vi "Param Test.vi"() -> ()   [LabVIEW 2020]
uses:
  g_ar_toolkit.capture/CameraStream/Camera Automatic Parameter Mode.ctl
  g_ar_toolkit.capture/CameraStream/Camera Parameter Information.ctl
  g_ar_toolkit.capture/CameraStream/CameraStream.lvclass/CameraStream.ctl
  g_ar_toolkit.image/CreateEmptyImageARGB.vi
  g_ar_toolkit.image/DrawImageToPictureARGB.vi
  7a086690-3a27-4eb0-92c0-07a8b9dc1a9d.vi
  bd8472f0-af5e-3fd8-803b-1528c88fa43f.vi
  g_ar_toolkit.capture/CameraStream/Get Focus Parameter Info.vi
  g_ar_toolkit.capture/CameraStream/Get Focus Parameter.vi
  g_ar_toolkit.capture/CameraStream/Get Zoom Parameter Info.vi
  g_ar_toolkit.capture/CameraStream/Get Zoom Parameter.vi
  g_ar_toolkit.capture/CameraStream/Get White Balance Parameter Info.vi
  g_ar_toolkit.capture/CameraStream/Get White Balance Parameter.vi
  g_ar_toolkit.capture/CameraStream/Get Brightenss Parameter Info.vi
  g_ar_toolkit.capture/CameraStream/Get Brightenss Parameter.vi
  g_ar_toolkit.capture/CameraStream/Get Contrast Parameter Info.vi
  g_ar_toolkit.capture/CameraStream/Get Contrast Parameter.vi
  g_ar_toolkit.capture/CameraStream/Get Saturation Parameter Info.vi
  g_ar_toolkit.capture/CameraStream/Get Saturation Parameter.vi
  g_ar_toolkit.capture/CameraStream/Get Gamma Parameter Info.vi
  g_ar_toolkit.capture/CameraStream/Get Gamma Parameter.vi
  g_ar_toolkit.capture/CameraStream/Get Hue Parameter Info.vi
  g_ar_toolkit.capture/CameraStream/Get Hue Parameter.vi
  g_ar_toolkit.capture/CameraStream/Get Sharpness Parameter Info.vi
  g_ar_toolkit.capture/CameraStream/Get Sharpness Parameter.vi
  g_ar_toolkit.capture/CameraStream/Get Backlight Compensation Parameter Info.vi
  g_ar_toolkit.capture/CameraStream/Get Backlight Compensation Parameter.vi
  g_ar_toolkit.capture/CameraStream/Get Powerline Frequency Parameter Info.vi
  g_ar_toolkit.capture/CameraStream/Get Powerline Frequency Parameter.vi
  g_ar_toolkit.capture/CameraStream/Get Exposure Parameter Info.vi
  g_ar_toolkit.capture/CameraStream/Get Exposure Parameter.vi
  g_ar_toolkit.capture/CameraStream/Get Automatic Focus Mode.vi
  g_ar_toolkit.capture/CameraStream/Get Automatic White Balance Mode.vi
  g_ar_toolkit.capture/CameraStream/Get Automatic Gain Mode.vi
  g_ar_toolkit.capture/CameraStream/Get Automatic Exposure Mode.vi
  g_ar_toolkit.capture/CameraStream/Get Gain Parameter Info.vi
  g_ar_toolkit.capture/CameraStream/Get Gain Parameter.vi
  g_ar_toolkit.capture/CameraStream/Set Focus Parameter.vi
  g_ar_toolkit.capture/CameraStream/Set Zoom Parameter.vi
  g_ar_toolkit.capture/CameraStream/Set White Balance Parameter.vi
  g_ar_toolkit.capture/CameraStream/Set Gain Parameter.vi
  g_ar_toolkit.capture/CameraStream/Set Brightenss Parameter.vi
  g_ar_toolkit.capture/CameraStream/Set Contrast Parameter.vi
  g_ar_toolkit.capture/CameraStream/Set Saturation Parameter.vi
  g_ar_toolkit.capture/CameraStream/Set Gamma Parameter.vi
  g_ar_toolkit.capture/CameraStream/Set Hue Parameter.vi
  g_ar_toolkit.capture/CameraStream/Set Sharpness Parameter.vi
  g_ar_toolkit.capture/CameraStream/Set Backlight Compensation Parameter.vi
  g_ar_toolkit.capture/CameraStream/Set Powerline Frequency Parameter.vi
  g_ar_toolkit.capture/CameraStream/Set Exposure Parameter.vi
  g_ar_toolkit.capture/CameraStream/Set Automatic Focus Mode.vi.vi
  g_ar_toolkit.capture/CameraStream/Set Automatic White Balance Mode.vi
  g_ar_toolkit.capture/CameraStream/Set Automatic Gain Mode.vi.vi
  g_ar_toolkit.capture/CameraStream/Set Automatic Exposure Mode.vi.vi
  g_ar_toolkit.image/CreateEmptyImageARGB.vi/3321fa97-f432-4e1e-8db9-a0df79aed21b.vi
  g_ar_toolkit.image/DrawImageToPictureARGB.vi/8cd07b1b-062e-4fe4-9e87-2eb3dc89fe0e.vi
  g_ar_toolkit.capture/CameraStream/GetParameterInfo.vi
  g_ar_toolkit.capture/CameraStream/GetParameter.vi
  g_ar_toolkit.capture/CameraStream/GetAutomaticParameterMode.vi
  g_ar_toolkit.capture/CameraStream/SetParameter.vi
  g_ar_toolkit.capture/CameraStream/SetAutomaticParameterMode.vi
  g_ar_toolkit.image/ARGBColourToU32.vi
  <vilib>/Utility/error.llb/Error Cluster From Error Code.vi
  g_ar_toolkit.capture/CameraStream/CameraStream.lvclass
  g_ar_toolkit.capture/CameraManager/CameraManager.lvclass
  g_ar_toolkit.image/g_ar_toolkit.image.lvlib
panel:
  in  "Start/Stop":bool
  in  "Format":string(combo)
  in  "Source":string(combo)
  in  "Enumerate":bool
  in  "Erase":bool
  in  "Picture Zoom":dbl=1.0 min=0.0001 max=10.0 step=0.1
  out "Array":T2(array[cluster])
  in  "Automatic Parameter Mode":T3
  out "Array 2":T4(array[cluster])
  in  "Auto Parameter":T5(ring)
  out "Set Value":i32
  in  "enum":T6(ring)
  in  "Dial":i32(knob) step=1 scale=2800.0..6500.0
  out "2D Picture":picture
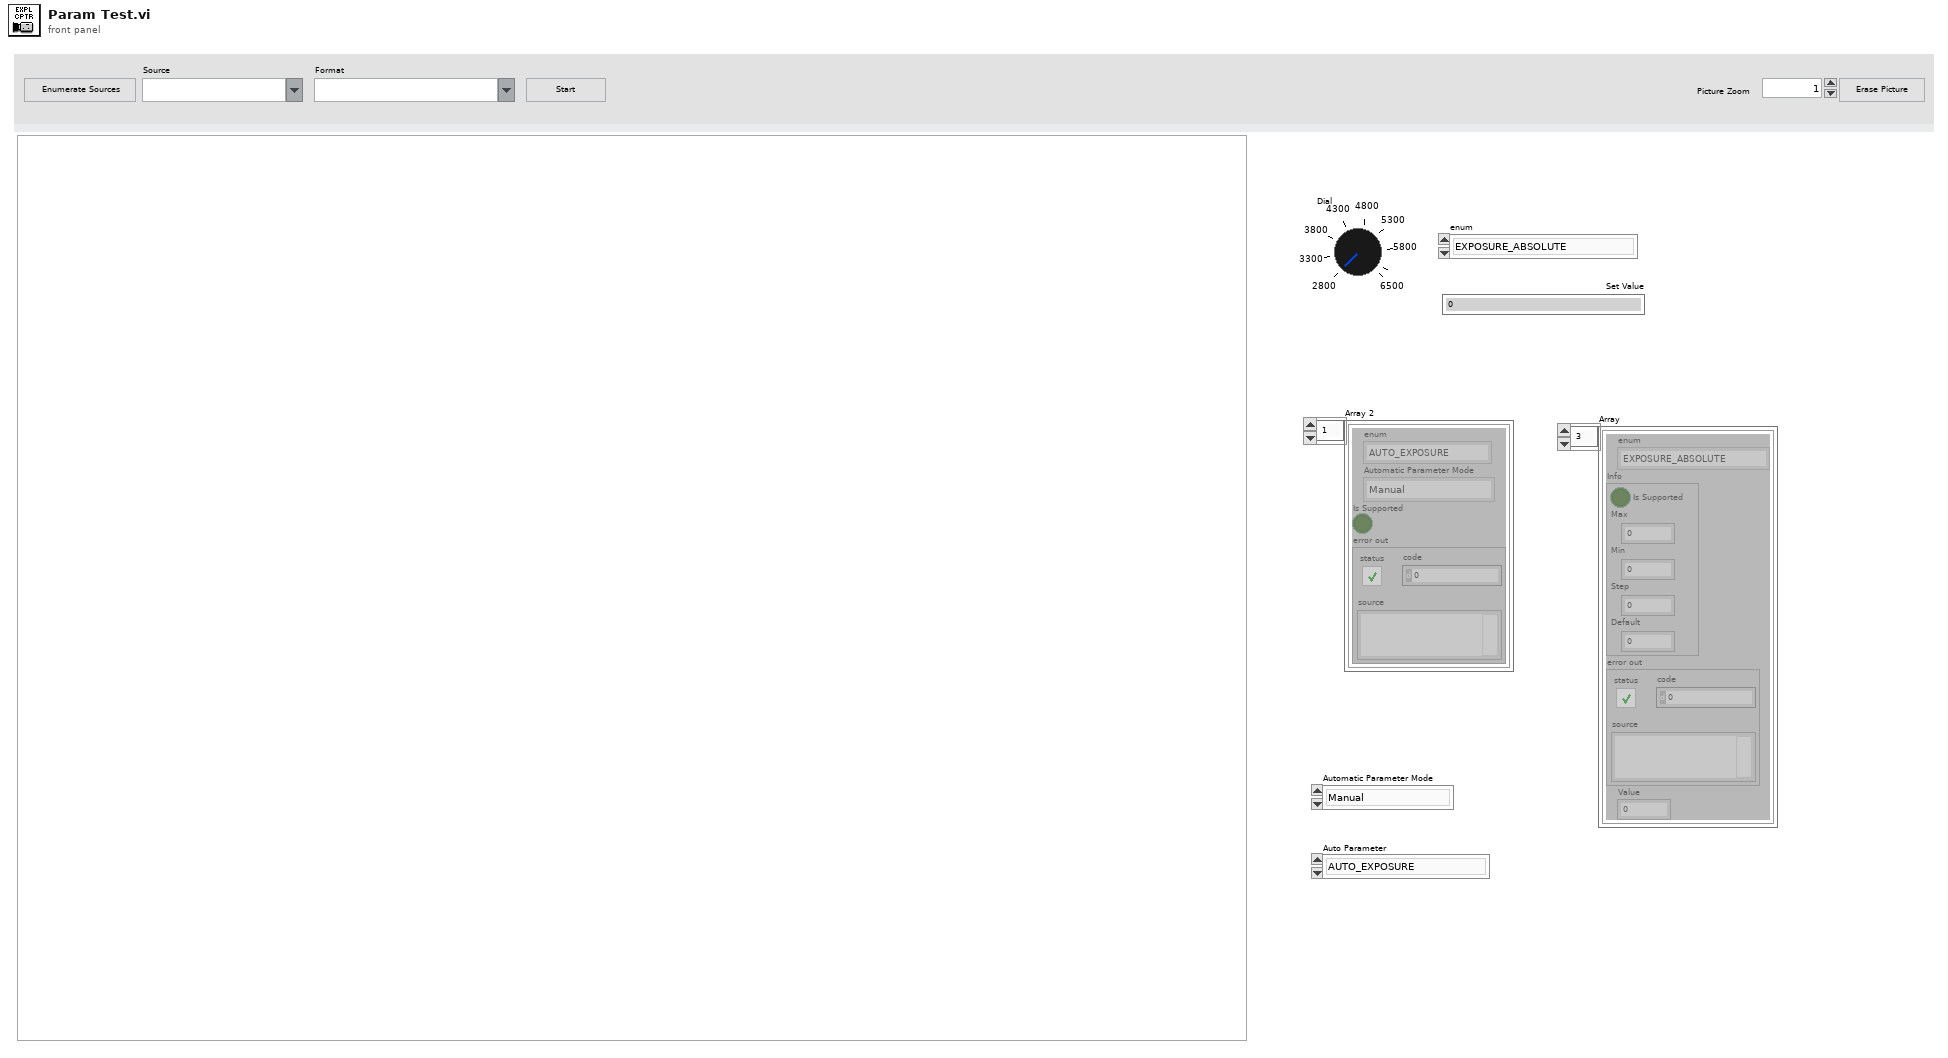
[diagram p1: front panel]
types:
  T1 = typedef "g_ar_toolkit.capture.lvlib/CameraStream.lvclass/Camera Parameter Information.ctl" = cluster{"Is Supported":bool, "Max":i32, "Min":i32, "Step":i32, "Default":i32}
  T2 = cluster{"enum":enum8{"EXPOSURE_ABSOLUTE", "FOCUS_ABSOLUTE", "ZOOM_ABSOLUTE", "WHITE_BALANCE_TEMPERATURE", "BRIGHTNESS", "CONTRAST", "SATURATION", "GAMMA", "HUE", "SHARPNESS", "BACKLIGHT_COMPENSATION", "POWER_LINE_FREQUENCY"}, "Info":T1, "error out":errorcluster, "Value":i32}[]
  T3 = typedef "g_ar_toolkit.capture.lvlib/CameraStream.lvclass/Camera Automatic Parameter Mode.ctl" = enum16{"Manual", "Automatic"}
  T4 = cluster{"enum":enum16{"AUTO_EXPOSURE", "AUTO_FOCUS", "AUTO_WHITEBALANCE", "AUTO_GAIN"}, "Automatic Parameter Mode":T3, "Is Supported":bool, "error out":errorcluster}[]
  T5 = enum16{"AUTO_EXPOSURE", "AUTO_FOCUS", "AUTO_WHITEBALANCE", "AUTO_GAIN"}
  T6 = enum8{"EXPOSURE_ABSOLUTE", "FOCUS_ABSOLUTE", "ZOOM_ABSOLUTE", "GAIN", "WHITE_BALANCE_TEMPERATURE", "BRIGHTNESS", "CONTRAST", "SATURATION", "GAMMA", "HUE", "SHARPNESS", "BACKLIGHT_COMPENSATION", "POWER_LINE_FREQUENCY"}
  T7 = enum8{"Enabled", "Disabled", "Disabled and Grayed Out"}
  T8 = enum8{"EXPOSURE_ABSOLUTE", "FOCUS_ABSOLUTE", "ZOOM_ABSOLUTE", "WHITE_BALANCE_TEMPERATURE", "BRIGHTNESS", "CONTRAST", "SATURATION", "GAMMA", "HUE", "SHARPNESS", "BACKLIGHT_COMPENSATION", "POWER_LINE_FREQUENCY"}
  T9 = typedef "g_ar_toolkit.capture.lvlib/CameraManager.lvclass/Device Enumeration.ctl" = cluster{"Name":string, "Streams":set{T10}}
  T10 = typedef "g_ar_toolkit.capture.lvlib/CameraManager.lvclass/Stream Parameters.ctl" = cluster{"Width":u16, "Height":u16, "FPS":u8}
  T11 = enum8{"EXPOSURE_ABSOLUTE", "FOCUS_ABSOLUTE", "ZOOM_ABSOLUTE", "WHITE_BALANCE_TEMPERATURE", "BRIGHTNESS", "CONTRAST", "SATURATION", "GAMMA", "HUE", "SHARPNESS", "BACKLIGHT_COMPENSATION", "POWER_LINE_FREQUENCY"}[]
  T12 = cluster{"enum":enum8{"EXPOSURE_ABSOLUTE", "FOCUS_ABSOLUTE", "ZOOM_ABSOLUTE", "WHITE_BALANCE_TEMPERATURE", "BRIGHTNESS", "CONTRAST", "SATURATION", "GAMMA", "HUE", "SHARPNESS", "BACKLIGHT_COMPENSATION", "POWER_LINE_FREQUENCY"}, "Info":T1, "error out":errorcluster, "Value":i32}
  T13 = enum16{"AUTO_EXPOSURE", "AUTO_FOCUS", "AUTO_WHITEBALANCE", "AUTO_GAIN"}[]
  T14 = cluster{"enum":enum16{"AUTO_EXPOSURE", "AUTO_FOCUS", "AUTO_WHITEBALANCE", "AUTO_GAIN"}, "Automatic Parameter Mode":T3, "Is Supported":bool, "error out":errorcluster}
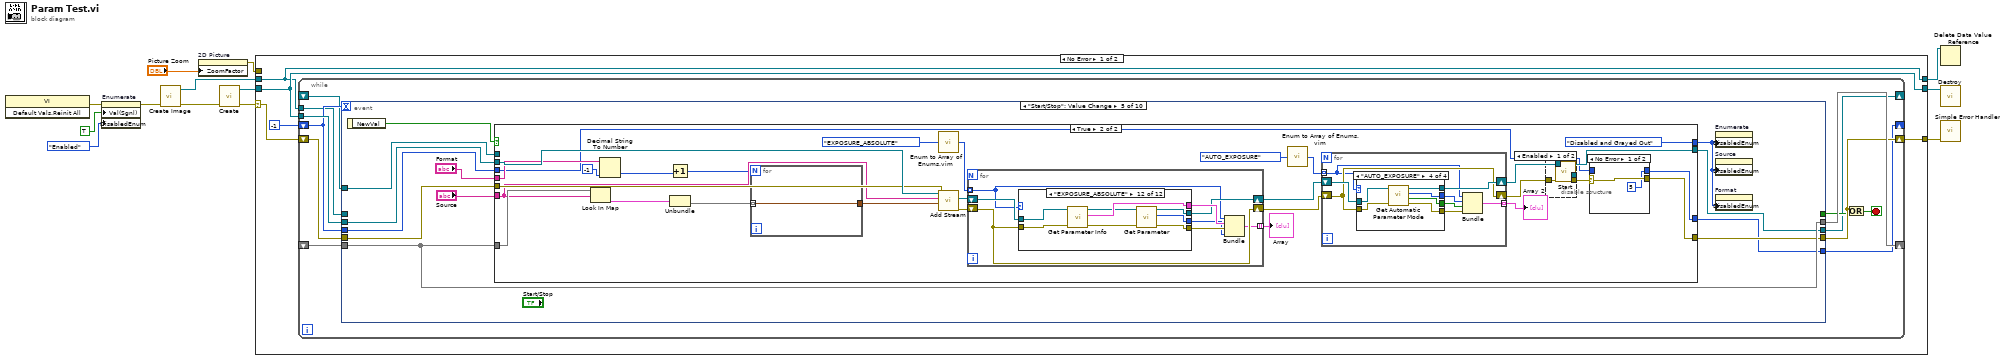
[diagram p0: block diagram]
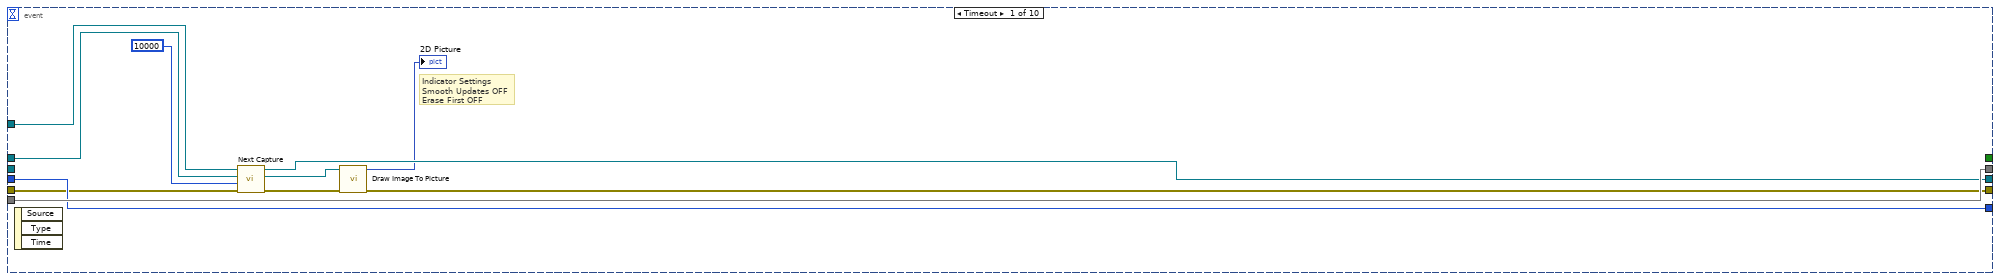
[diagram p2: hidden frame]
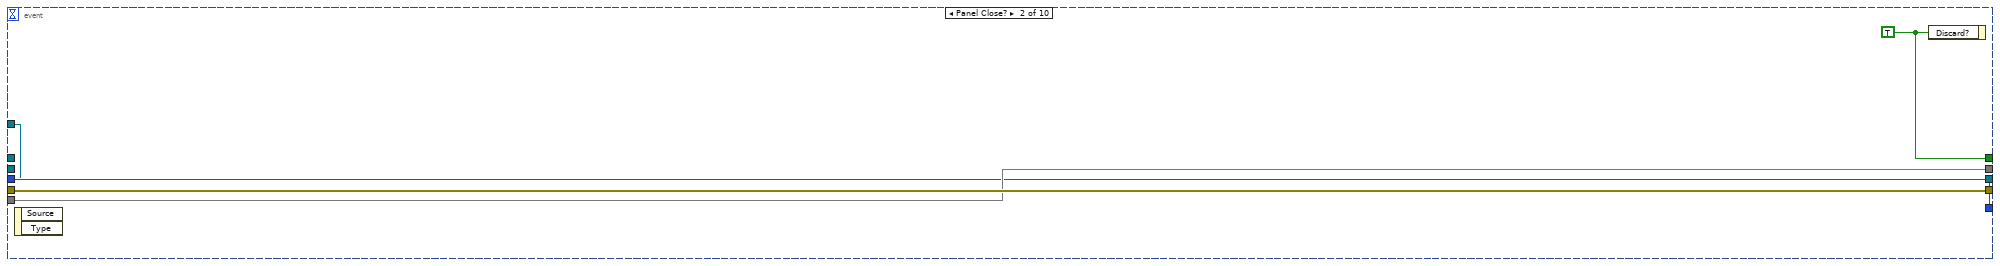
[diagram p3: hidden frame]
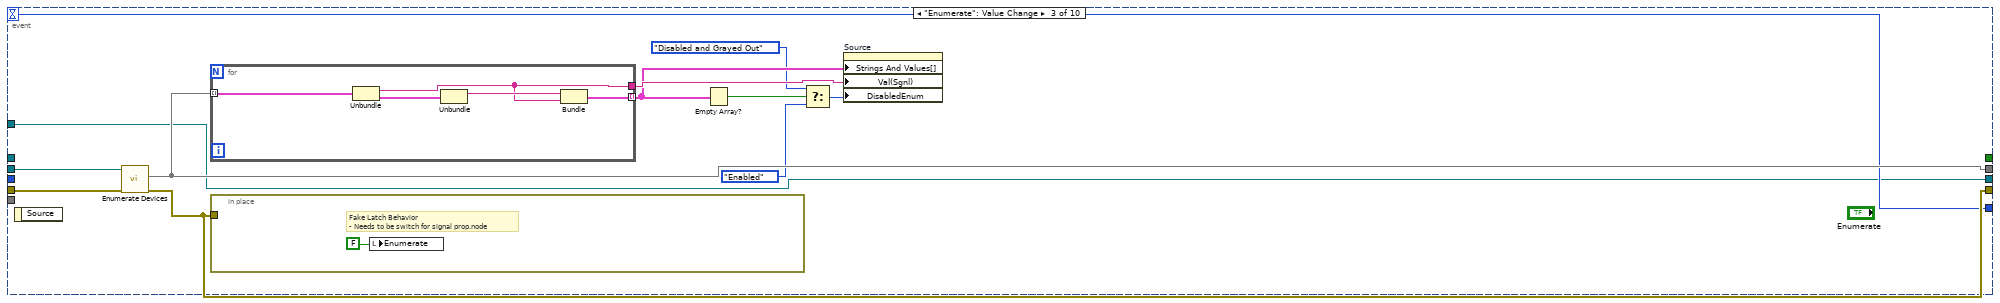
[diagram p4: hidden frame]
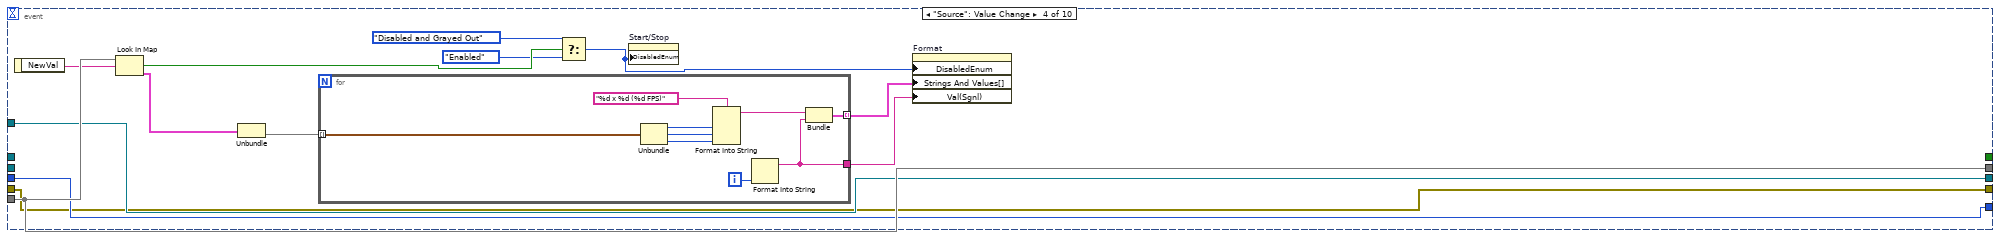
[diagram p5: hidden frame]
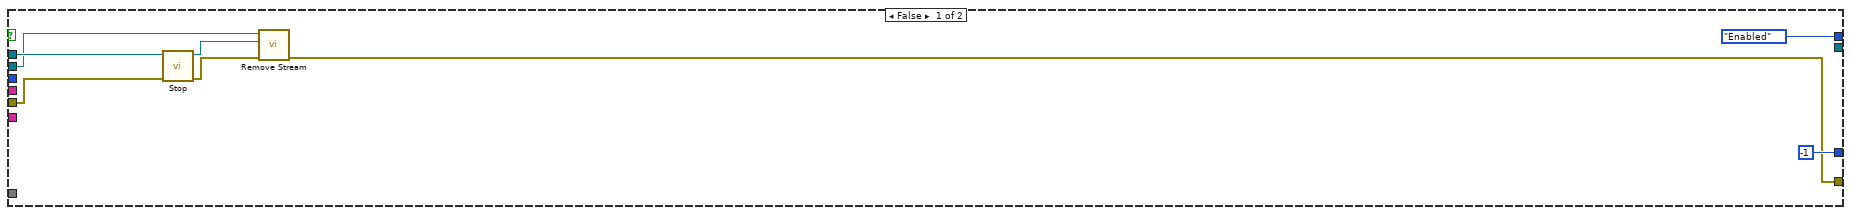
[diagram p6: hidden frame]
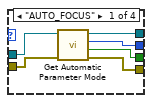
[diagram p8: hidden frame]
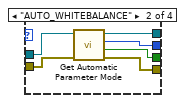
[diagram p9: hidden frame]
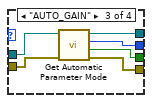
[diagram p10: hidden frame]
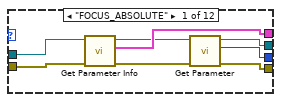
[diagram p11: hidden frame]
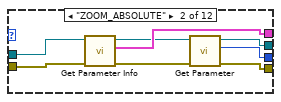
[diagram p12: hidden frame]
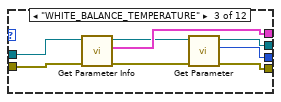
[diagram p13: hidden frame]
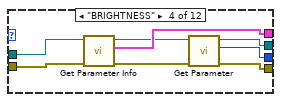
[diagram p14: hidden frame]
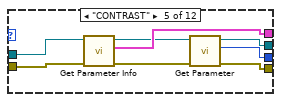
[diagram p15: hidden frame]
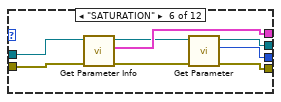
[diagram p16: hidden frame]
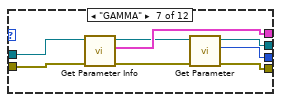
[diagram p17: hidden frame]
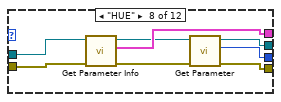
[diagram p18: hidden frame]
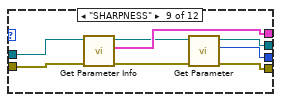
[diagram p19: hidden frame]
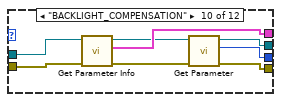
[diagram p20: hidden frame]
diagram:
  n1 = invoke class="VI" method="Default Vals.Reinit All"() -> (error out=w5:errorcluster)  [unwired: 3 in, 2 out]
  n2 = property on="Enumerate" class="Bool (strict)"(error in=w5, "Val(Sgnl)"=TRUE ("Value (Signaling)"), "DisabledEnum"=T7."Enabled" ("Disabled")) -> (error out=w1:errorcluster)  [unwired: 1 in, 1 out]
  n3 = call-poly "Create Image.vi"("error in (no error)"=w1) -> ("error out"=w4:errorcluster, "New ARGB Image"=w10:refnum<data-value>)  [unwired: 9 in]
  n4 = property on="2D Picture" class="Pict"("ZoomFactor"="Picture Zoom") -> (error out=w9:errorcluster)  [unwired: 2 in, 1 out]
  n5 = call "Create.vi"("error in (no error)"=w4) -> ("error out"=w13:errorcluster, "CameraManager"=w2:refnum<data-value>)  [unwired: 9 in]
  n6 = case shown="No Error" w13 {
    selector: w13 -> [w18 w564]
    tunnel: w2 -> [w17 w566]
    tunnel: [w17 w566] -> w12
    tunnel: w10 -> [w15 w565]
    tunnel: w9 -> [_ _]
    tunnel: [w15 w565] -> w7
    tunnel: [w14 w564] -> w6
    frame No Error {
      n7 = while {
        tunnel: w17 -> [w30]
        shift-right: [w28] -> _
        shift-left: _ -> [w27]
        shift-right: [w26] -> w14
        shift-left: w18 -> [w29]
        shift-right: [w23] -> _
        shift-left: -1 -> [w22]
        shift-right: [w21] -> _
        shift-left: _ -> [w20]
        tunnel: w15 -> [w19]
        stop <- w25 stop-if-true
        n8 = event shown="[4] \"Start/Stop\": Value Change" {
          selector: _ -> [_ _ _ _ _ _ _ _ _ _]
          dyn-events: _ -> [_ _ _ _ _ _ _ _ _ _]
          timeout: w22 -> [_ _ w53 _ _ _ _ _ _ _]
          tunnel: w30 -> [_ _ w58 _ w94 _ _ _ _ _]
          tunnel: w29 -> [w33 w45 w57 w65 w95 w287 w442 w527 w554 w560]
          tunnel: [w41 w44 w56 w77 w93 w299 w446 w532 w557 w558] -> w28
          tunnel: w27 -> [w41 w44 _ w77 w93 w299 w446 w532 w557 w558]
          tunnel: [w32 w45 w54 w65 w92 w289 w441 w528 w554 w559] -> w26
          tunnel: [_ w46 _ _ _ _ _ _ _ _] -> w24
          tunnel: [w40 w43 w53 w67 w89 w298 w445 w531 w556 w563] -> w23
          tunnel: w22 -> [w40 w43 _ w67 w90 w298 w445 w531 w556 w563]
          tunnel: [w38 w42 w52 w66 w91 w290 w443 w529 w555 w562] -> w21
          tunnel: w20 -> [w39 w42 w52 w66 w88 w288 w444 w530 w555 w562]
          tunnel: w19 -> [w37 _ _ _ _ _ _ _ _ _]
          event Timeout {
            # "Indicator Settings\nSmooth Updates OFF\nErase First OFF"
            n9 = event-data() -> ()  [unwired: 1 in, 3 out]
            n10 = call "Next Capture.vi"("error in (no error)"=w33, "timeout (ms)"=u16 10000, "ARGB Image Destination"=w37, "Stream"=w39) -> ("error out"=w34:errorcluster, "ARGB Image (duplicate)"=w35:refnum<data-value>, "Stream (duplicate)"=w38:refnum<data-value>)  [unwired: 5 in]
            n11 = call-poly "Draw Image To Picture.vi"("error in (no error)"=w34, "ARGB Image Source"=w35) -> ("error out"=w32:errorcluster, "Picture"=→"2D Picture":picture)  [unwired: 8 in]
          }
          event Panel Close? {
            w46 = TRUE ("Discard?")
            n12 = event-data() -> ()  [unwired: 1 in, 2 out]
            n13 = event-data("Discard?"=w46) -> ()  [unwired: 1 in, 1 out]
          }
          event "Enumerate": Value Change {
            n14 = event-data() -> ()  [unwired: 1 in, 1 out]
            n15 = call "Enumerate Devices.vi"("error in (no error)"=w57, "CameraManager"=w58) -> ("error out"=w54:errorcluster, "Devices"=w56:map{string, T9})  [unwired: 7 in, 1 out]
            n16 = for {
              tunnel: w56 -> [w64] mode=indexing
              tunnel: [w61] -> w50 mode=indexing
              tunnel: [w60] -> w55
              n17 = Unbundle(w64) -> ("id"=w60:string, "Info"=w63:T9)
              n18 = Unbundle(w63) -> ("Name"=w62:string)  [unwired: 1 out]
              n19 = Bundle("Name"=w62, "id"=w60) -> (w61:cluster{"Name":string, "id":string})  [unwired: 1 in]
            }
            n20 = in-place {
              in-place-border: w54 -> [_]
              # "Fake Latch Behavior\n- Needs to be switch for signal prop.node"
              n21 = local write "Enumerate"(FALSE ("Re-Enumerate Sources")) -> ()
            }
            n22 = Empty Array?(array=w50) -> (empty?=w51:bool)
            n23 = Select(t=T7."Disabled and Grayed Out", s=w51, f=T7."Enabled" ("Disabled")) -> (s? t:f=w47:T7)
            n24 = property on="Source" class="CmbBox"("Strings And Values[]"=w50, "Val(Sgnl)"=w55, "DisabledEnum"=w47) -> ()  [unwired: 2 in, 2 out]
          }
          event "Source": Value Change {
            n25 = event-data() -> ("NewVal"=w76:string)  [unwired: 1 in]
            n26 = Look In Map(map=w77, key=w76) -> (key not found?=w75:bool, value=w72:T9)  [unwired: 1 in]
            n27 = Unbundle(w72) -> ("Streams"=w71:set{T10})  [unwired: 1 out]
            n28 = for {
              tunnel: w71 -> [w81] mode=indexing
              tunnel: [w84] -> w69 mode=indexing
              tunnel: [w83] -> w68
              i -> [w86]
              n29 = Unbundle(w81) -> ("Width"=w80:u16, "Height"=w79:u16, "FPS"=w78:u8)
              n30 = Format Into String(format string="%d x %d (%d FPS)", w80, w79, w78) -> (resulting string=w85:string)  [unwired: 2 in, 1 out]
              n31 = Format Into String(w86) -> (resulting string=w83:string)  [unwired: 3 in, 1 out]
              n32 = Bundle(w85, w83) -> (w84:cluster{string, string})  [unwired: 1 in]
            }
            n33 = Select(t=T7."Disabled and Grayed Out" ("Disabled"), s=w75, f=T7."Enabled") -> (s? t:f=w70:T7)
            n34 = property on="Start/Stop" class="Bool (strict)"("DisabledEnum"=w70) -> ()  [unwired: 2 in, 2 out]
            n35 = property on="Format" class="CmbBox"("DisabledEnum"=w70, "Strings And Values[]"=w69, "Val(Sgnl)"=w68) -> ()  [unwired: 2 in, 2 out]
          }
          event "Start/Stop": Value Change {
            n36 = event-data() -> ("NewVal"=w98:bool)  [unwired: 1 in]
            n37 = case shown="True" w98 {
              tunnel: "Source" -> [_ w131]
              tunnel: "Format" -> [_ w130]
              tunnel: w95 -> [w103 w134]
              tunnel: w94 -> [w105 w135]
              tunnel: w93 -> [_ w133]
              tunnel: [w100 w125] -> w92
              tunnel: [_ w123] -> w91
              tunnel: w90 -> [_ w122]
              tunnel: [-1 w121] -> w89
              tunnel: w88 -> [w106 _]
              tunnel: [T7."Enabled" ("Disabled") T7."Disabled and Grayed Out" ("Disabled")] -> w87
              frame False {
                n38 = call "Stop.vi"("error in (no error)"=w103, "Stream"=w106) -> ("error out"=w102:errorcluster, "Stream (duplicate)"=w104:refnum<data-value>)  [unwired: 8 in]
                n39 = call "Remove Stream.vi"("error in (no error)"=w102, "Stream"=w104, "CameraManager"=w105) -> ("error out"=w100:errorcluster)  [unwired: 7 in, 1 out]
              }
              frame True {
                n40 = Look In Map(map=w133, key=w131) -> (value=w132:T9)  [unwired: 1 in, 1 out]
                n41 = Decimal String To Number(string=w130, default (0L)=-1 ("default (0 I32)")) -> (number=w126:i32)  [unwired: 1 in, 1 out]
                n42 = Increment(x=w126) -> (x+1=w127:i32)
                n43 = Unbundle(w132) -> ("Streams"=w129:set{T10})  [unwired: 1 out]
                n44 = for {
                  N: w127 -> [_]
                  tunnel: w129 -> [w282] mode=indexing
                  tunnel: [w282] -> w118
                }
                n45 = call "Enum to Array of Enums.vim"("enum"=T8."EXPOSURE_ABSOLUTE" ("Camera Parameter")) -> ("array of enums"=w115:T11)
                n46 = call "Add Stream.vi"("error in (no error)"=w134, "Desired Stream Parameters"=w118, "Device ID"=w131, "CameraManager"=w135) -> ("error out"=w120:errorcluster, "Stream"=w117:refnum<data-value>)  [unwired: 5 in, 1 out]
                n47 = for {
                  shift-right: [w180] -> w113
                  shift-left: w120 -> [w180]
                  shift-right: [w176] -> w114
                  shift-left: w117 -> [w181]
                  tunnel: w115 -> [w174] mode=indexing
                  tunnel: [w179] -> w107 mode=indexing
                  n48 = case shown="\"EXPOSURE_ABSOLUTE\"" w174 {
                    tunnel: w181 -> [w189 w197 w205 w213 w221 w229 w237 w245 w253 w261 w269 w277]
                    tunnel: w180 -> [w188 w196 w204 w212 w220 w228 w236 w244 w252 w260 w268 w276]
                    tunnel: [w186 w194 w202 w210 w218 w226 w234 w242 w250 w258 w266 w274] -> w178
                    tunnel: [w185 w193 w201 w209 w217 w225 w233 w241 w249 w257 w265 w273] -> w177
                    tunnel: [w183 w191 w199 w207 w215 w223 w231 w239 w247 w255 w263 w271] -> w176
                    tunnel: [w182 w190 w198 w206 w214 w222 w230 w238 w246 w254 w262 w270] -> w175
                    frame "FOCUS_ABSOLUTE" {
                      n49 = call-poly "Get Parameter Info.vi"("error in (no error)"=w188, "Stream"=w189) -> ("error out"=w187:errorcluster, "Info"=w186:T1, "Stream (duplicate)"=w184:refnum<data-value>)  [unwired: 7 in]
                      n50 = call-poly "Get Parameter.vi"("error in (no error)"=w187, "Stream"=w184) -> ("error out"=w185:errorcluster, "Value"=w182:i32, "Stream (duplicate)"=w183:refnum<data-value>)  [unwired: 7 in]
                    }
                    frame "ZOOM_ABSOLUTE" {
                      n51 = call-poly "Get Parameter Info.vi"("error in (no error)"=w196, "Stream"=w197) -> ("error out"=w195:errorcluster, "Info"=w194:T1, "Stream (duplicate)"=w192:refnum<data-value>)  [unwired: 7 in]
                      n52 = call-poly "Get Parameter.vi"("error in (no error)"=w195, "Stream"=w192) -> ("error out"=w193:errorcluster, "Value"=w190:i32, "Stream (duplicate)"=w191:refnum<data-value>)  [unwired: 7 in]
                    }
                    frame "WHITE_BALANCE_TEMPERATURE" {
                      n53 = call-poly "Get Parameter Info.vi"("error in (no error)"=w204, "Stream"=w205) -> ("error out"=w203:errorcluster, "Info"=w202:T1, "Stream (duplicate)"=w200:refnum<data-value>)  [unwired: 7 in]
                      n54 = call-poly "Get Parameter.vi"("error in (no error)"=w203, "Stream"=w200) -> ("error out"=w201:errorcluster, "Value"=w198:i32, "Stream (duplicate)"=w199:refnum<data-value>)  [unwired: 7 in]
                    }
                    frame "BRIGHTNESS" {
                      n55 = call-poly "Get Parameter Info.vi"("error in (no error)"=w212, "Stream"=w213) -> ("error out"=w211:errorcluster, "Info"=w210:T1, "Stream (duplicate)"=w208:refnum<data-value>)  [unwired: 7 in]
                      n56 = call-poly "Get Parameter.vi"("error in (no error)"=w211, "Stream"=w208) -> ("error out"=w209:errorcluster, "Value"=w206:i32, "Stream (duplicate)"=w207:refnum<data-value>)  [unwired: 7 in]
                    }
                    frame "CONTRAST" {
                      n57 = call-poly "Get Parameter Info.vi"("error in (no error)"=w220, "Stream"=w221) -> ("error out"=w219:errorcluster, "Info"=w218:T1, "Stream (duplicate)"=w216:refnum<data-value>)  [unwired: 7 in]
                      n58 = call-poly "Get Parameter.vi"("error in (no error)"=w219, "Stream"=w216) -> ("error out"=w217:errorcluster, "Value"=w214:i32, "Stream (duplicate)"=w215:refnum<data-value>)  [unwired: 7 in]
                    }
                    frame "SATURATION" {
                      n59 = call-poly "Get Parameter Info.vi"("error in (no error)"=w228, "Stream"=w229) -> ("error out"=w227:errorcluster, "Info"=w226:T1, "Stream (duplicate)"=w224:refnum<data-value>)  [unwired: 7 in]
                      n60 = call-poly "Get Parameter.vi"("error in (no error)"=w227, "Stream"=w224) -> ("error out"=w225:errorcluster, "Value"=w222:i32, "Stream (duplicate)"=w223:refnum<data-value>)  [unwired: 7 in]
                    }
                    frame "GAMMA" {
                      n61 = call-poly "Get Parameter Info.vi"("error in (no error)"=w236, "Stream"=w237) -> ("error out"=w235:errorcluster, "Info"=w234:T1, "Stream (duplicate)"=w232:refnum<data-value>)  [unwired: 7 in]
                      n62 = call-poly "Get Parameter.vi"("error in (no error)"=w235, "Stream"=w232) -> ("error out"=w233:errorcluster, "Value"=w230:i32, "Stream (duplicate)"=w231:refnum<data-value>)  [unwired: 7 in]
                    }
                    frame "HUE" {
                      n63 = call-poly "Get Parameter Info.vi"("error in (no error)"=w244, "Stream"=w245) -> ("error out"=w243:errorcluster, "Info"=w242:T1, "Stream (duplicate)"=w240:refnum<data-value>)  [unwired: 7 in]
                      n64 = call-poly "Get Parameter.vi"("error in (no error)"=w243, "Stream"=w240) -> ("error out"=w241:errorcluster, "Value"=w238:i32, "Stream (duplicate)"=w239:refnum<data-value>)  [unwired: 7 in]
                    }
                    frame "SHARPNESS" {
                      n65 = call-poly "Get Parameter Info.vi"("error in (no error)"=w252, "Stream"=w253) -> ("error out"=w251:errorcluster, "Info"=w250:T1, "Stream (duplicate)"=w248:refnum<data-value>)  [unwired: 7 in]
                      n66 = call-poly "Get Parameter.vi"("error in (no error)"=w251, "Stream"=w248) -> ("error out"=w249:errorcluster, "Value"=w246:i32, "Stream (duplicate)"=w247:refnum<data-value>)  [unwired: 7 in]
                    }
                    frame "BACKLIGHT_COMPENSATION" {
                      n67 = call-poly "Get Parameter Info.vi"("error in (no error)"=w260, "Stream"=w261) -> ("error out"=w259:errorcluster, "Info"=w258:T1, "Stream (duplicate)"=w256:refnum<data-value>)  [unwired: 7 in]
                      n68 = call-poly "Get Parameter.vi"("error in (no error)"=w259, "Stream"=w256) -> ("error out"=w257:errorcluster, "Value"=w254:i32, "Stream (duplicate)"=w255:refnum<data-value>)  [unwired: 7 in]
                    }
                    frame "POWER_LINE_FREQUENCY" {
                      n69 = call-poly "Get Parameter Info.vi"("error in (no error)"=w268, "Stream"=w269) -> ("error out"=w267:errorcluster, "Info"=w266:T1, "Stream (duplicate)"=w264:refnum<data-value>)  [unwired: 7 in]
                      n70 = call-poly "Get Parameter.vi"("error in (no error)"=w267, "Stream"=w264) -> ("error out"=w265:errorcluster, "Value"=w262:i32, "Stream (duplicate)"=w263:refnum<data-value>)  [unwired: 7 in]
                    }
                    frame "EXPOSURE_ABSOLUTE" {
                      n71 = call-poly "Get Parameter Info.vi"("error in (no error)"=w276, "Stream"=w277) -> ("error out"=w275:errorcluster, "Info"=w274:T1, "Stream (duplicate)"=w272:refnum<data-value>)  [unwired: 7 in]
                      n72 = call-poly "Get Parameter.vi"("error in (no error)"=w275, "Stream"=w272) -> ("error out"=w273:errorcluster, "Value"=w270:i32, "Stream (duplicate)"=w271:refnum<data-value>)  [unwired: 7 in]
                    }
                  }
                  n73 = Bundle("enum"=w174, "Info"=w178, "error out"=w177, "Value"=w175) -> (w179:T12)  [unwired: 1 in]
                }
                "Array" <- w107
                n74 = call "Enum to Array of Enums.vim"("enum"=T5."AUTO_EXPOSURE" ("Auto Parameter")) -> ("array of enums"=w109:T13)
                n75 = for {
                  shift-right: [w145] -> w112
                  shift-left: w113 -> [w145]
                  shift-right: [w147] -> w111
                  shift-left: w114 -> [w149]
                  tunnel: [w148] -> w108 mode=indexing
                  tunnel: w109 -> [w142] mode=indexing
                  n76 = case shown="\"AUTO_EXPOSURE\"" w142 {
                    tunnel: w149 -> [w155 w161 w167 w173]
                    tunnel: [w154 w160 w166 w172] -> w147
                    tunnel: [w153 w159 w165 w171] -> w146
                    tunnel: w145 -> [w152 w158 w164 w170]
                    tunnel: [w151 w157 w163 w169] -> w144
                    tunnel: [w150 w156 w162 w168] -> w143
                    frame "AUTO_FOCUS" {
                      n77 = call-poly "Get Automatic Parameter Mode.vi"("error in (no error)"=w152, "Stream"=w155) -> ("error out"=w153:errorcluster, "Is Supported"=w150:bool, "Automatic Parameter Mode"=w151:T3, "Stream (duplicate)"=w154:refnum<data-value>)  [unwired: 6 in]
                    }
                    frame "AUTO_WHITEBALANCE" {
                      n78 = call-poly "Get Automatic Parameter Mode.vi"("error in (no error)"=w158, "Stream"=w161) -> ("error out"=w159:errorcluster, "Is Supported"=w156:bool, "Automatic Parameter Mode"=w157:T3, "Stream (duplicate)"=w160:refnum<data-value>)  [unwired: 6 in]
                    }
                    frame "AUTO_GAIN" {
                      n79 = call-poly "Get Automatic Parameter Mode.vi"("error in (no error)"=w164, "Stream"=w167) -> ("error out"=w165:errorcluster, "Is Supported"=w162:bool, "Automatic Parameter Mode"=w163:T3, "Stream (duplicate)"=w166:refnum<data-value>)  [unwired: 6 in]
                    }
                    frame "AUTO_EXPOSURE" {
                      n80 = call-poly "Get Automatic Parameter Mode.vi"("error in (no error)"=w170, "Stream"=w173) -> ("error out"=w171:errorcluster, "Is Supported"=w168:bool, "Automatic Parameter Mode"=w169:T3, "Stream (duplicate)"=w172:refnum<data-value>)  [unwired: 6 in]
                    }
                  }
                  n81 = Bundle("enum"=w142, "Automatic Parameter Mode"=w144, "Is Supported"=w143, "error out"=w146) -> (w148:T14)  [unwired: 1 in]
                }
                "Array 2" <- w108
                n82 = disable-structure shown="Enabled" {
                  disable-tunnel: [w139 w141] -> w124
                  disable-tunnel: [w138 w140] -> w123
                  disable-tunnel: w112 -> [w137 w141]
                  disable-tunnel: w111 -> [w136 w140]
                  frame Enabled {
                    n83 = call "Start.vi"("error in (no error)"=w137, "Stream"=w136) -> ("error out"=w139:errorcluster, "Stream (duplicate)"=w138:refnum<data-value>)  [unwired: 8 in]
                  }
                  frame Disabled {
                  }
                }
                n84 = case shown="No Error" w124 {
                  selector: w124 -> [w279 w280]
                  tunnel: [w279 w280] -> w125
                  tunnel: w122 -> [_ w281]
                  tunnel: [5 w281] -> w121
                  frame No Error {
                  }
                  frame Error {
                  }
                }
              }
            }
            n85 = property on="Enumerate" class="Bool (strict)"("DisabledEnum"=w87) -> ()  [unwired: 2 in, 2 out]
            n86 = property on="Source" class="CmbBox"("DisabledEnum"=w87) -> ()  [unwired: 2 in, 2 out]
            n87 = property on="Format" class="CmbBox"("DisabledEnum"=w87) -> ()  [unwired: 2 in, 2 out]
          }
          event "enum": Value Change {
            n88 = event-data() -> ("NewVal"=w283:T6)  [unwired: 1 in, 3 out]
            n89 = case shown="\"GAIN\"" w283 {
              tunnel: w288 -> [w304 w309 w314 w319 w324 w329 w334 w339 w344 w349 w354 w359 w364]
              tunnel: w287 -> [w303 w308 w313 w318 w323 w328 w333 w338 w343 w348 w353 w358 w363]
              tunnel: [w301 w306 w311 w316 w321 w326 w331 w336 w341 w346 w351 w356 w361] -> w284
              tunnel: [w302 w307 w312 w317 w322 w327 w332 w337 w342 w347 w352 w357 w362] -> w285
              tunnel: [w300 w305 w310 w315 w320 w325 w330 w335 w340 w345 w350 w355 w360] -> w286
              frame "FOCUS_ABSOLUTE" {
                n90 = call-poly "Get Parameter Info.vi"("error in (no error)"=w303, "Stream"=w304) -> ("error out"=w302:errorcluster, "Info"=w301:T1, "Stream (duplicate)"=w300:refnum<data-value>)  [unwired: 7 in]
              }
              frame "ZOOM_ABSOLUTE" {
                n91 = call-poly "Get Parameter Info.vi"("error in (no error)"=w308, "Stream"=w309) -> ("error out"=w307:errorcluster, "Info"=w306:T1, "Stream (duplicate)"=w305:refnum<data-value>)  [unwired: 7 in]
              }
              frame "WHITE_BALANCE_TEMPERATURE" {
                n92 = call-poly "Get Parameter Info.vi"("error in (no error)"=w313, "Stream"=w314) -> ("error out"=w312:errorcluster, "Info"=w311:T1, "Stream (duplicate)"=w310:refnum<data-value>)  [unwired: 7 in]
              }
              frame "GAIN" {
                n93 = call-poly "Get Parameter Info.vi"("error in (no error)"=w318, "Stream"=w319) -> ("error out"=w317:errorcluster, "Info"=w316:T1, "Stream (duplicate)"=w315:refnum<data-value>)  [unwired: 7 in]
              }
              frame "BRIGHTNESS" {
                n94 = call-poly "Get Parameter Info.vi"("error in (no error)"=w323, "Stream"=w324) -> ("error out"=w322:errorcluster, "Info"=w321:T1, "Stream (duplicate)"=w320:refnum<data-value>)  [unwired: 7 in]
              }
              frame "CONTRAST" {
                n95 = call-poly "Get Parameter Info.vi"("error in (no error)"=w328, "Stream"=w329) -> ("error out"=w327:errorcluster, "Info"=w326:T1, "Stream (duplicate)"=w325:refnum<data-value>)  [unwired: 7 in]
              }
              frame "SATURATION" {
                n96 = call-poly "Get Parameter Info.vi"("error in (no error)"=w333, "Stream"=w334) -> ("error out"=w332:errorcluster, "Info"=w331:T1, "Stream (duplicate)"=w330:refnum<data-value>)  [unwired: 7 in]
              }
              frame "GAMMA" {
                n97 = call-poly "Get Parameter Info.vi"("error in (no error)"=w338, "Stream"=w339) -> ("error out"=w337:errorcluster, "Info"=w336:T1, "Stream (duplicate)"=w335:refnum<data-value>)  [unwired: 7 in]
              }
              frame "HUE" {
                n98 = call-poly "Get Parameter Info.vi"("error in (no error)"=w343, "Stream"=w344) -> ("error out"=w342:errorcluster, "Info"=w341:T1, "Stream (duplicate)"=w340:refnum<data-value>)  [unwired: 7 in]
              }
              frame "SHARPNESS" {
                n99 = call-poly "Get Parameter Info.vi"("error in (no error)"=w348, "Stream"=w349) -> ("error out"=w347:errorcluster, "Info"=w346:T1, "Stream (duplicate)"=w345:refnum<data-value>)  [unwired: 7 in]
              }
              frame "BACKLIGHT_COMPENSATION" {
                n100 = call-poly "Get Parameter Info.vi"("error in (no error)"=w353, "Stream"=w354) -> ("error out"=w352:errorcluster, "Info"=w351:T1, "Stream (duplicate)"=w350:refnum<data-value>)  [unwired: 7 in]
              }
              frame "POWER_LINE_FREQUENCY" {
                n101 = call-poly "Get Parameter Info.vi"("error in (no error)"=w358, "Stream"=w359) -> ("error out"=w357:errorcluster, "Info"=w356:T1, "Stream (duplicate)"=w355:refnum<data-value>)  [unwired: 7 in]
              }
              frame "EXPOSURE_ABSOLUTE" {
                n102 = call-poly "Get Parameter Info.vi"("error in (no error)"=w363, "Stream"=w364) -> ("error out"=w362:errorcluster, "Info"=w361:T1, "Stream (duplicate)"=w360:refnum<data-value>)  [unwired: 7 in]
              }
            }
            n103 = Unbundle By Name(w284) -> ("Is Supported"=w291:bool, "Max"=w294:i32, "Min"=w293:i32, "Step"=w292:i32)  [unwired: 1 out]
            n104 = case shown="True" w291 {
              tunnel: [w366 w370] -> w290
              tunnel: w286 -> [w366 w372]
              tunnel: [w365 w369] -> w289
              tunnel: w285 -> [w365 w371]
              tunnel: w283 -> [_ w367]
              frame False {
              }
              frame True {
                n105 = case shown="\"GAIN\"" w367 {
                  tunnel: w372 -> [w377 w382 w387 w392 w397 w402 w407 w412 w417 w422 w427 w432 w437]
                  tunnel: w371 -> [w376 w381 w386 w391 w396 w401 w406 w411 w416 w421 w426 w431 w436]
                  tunnel: [w375 w380 w385 w390 w395 w400 w405 w410 w415 w420 w425 w430 w435] -> w369
                  tunnel: [w374 w379 w384 w389 w394 w399 w404 w409 w414 w419 w424 w429 w434] -> w370
                  tunnel: [w373 w378 w383 w388 w393 w398 w403 w408 w413 w418 w423 w428 w433] -> w368
                  frame "FOCUS_ABSOLUTE" {
                    n106 = call-poly "Get Parameter.vi"("error in (no error)"=w376, "Stream"=w377) -> ("error out"=w375:errorcluster, "Value"=w373:i32, "Stream (duplicate)"=w374:refnum<data-value>)  [unwired: 7 in]
                  }
                  frame "ZOOM_ABSOLUTE" {
                    n107 = call-poly "Get Parameter.vi"("error in (no error)"=w381, "Stream"=w382) -> ("error out"=w380:errorcluster, "Value"=w378:i32, "Stream (duplicate)"=w379:refnum<data-value>)  [unwired: 7 in]
                  }
                  frame "WHITE_BALANCE_TEMPERATURE" {
                    n108 = call-poly "Get Parameter.vi"("error in (no error)"=w386, "Stream"=w387) -> ("error out"=w385:errorcluster, "Value"=w383:i32, "Stream (duplicate)"=w384:refnum<data-value>)  [unwired: 7 in]
                  }
                  frame "GAIN" {
                    n109 = call-poly "Get Parameter.vi"("error in (no error)"=w391, "Stream"=w392) -> ("error out"=w390:errorcluster, "Value"=w388:i32, "Stream (duplicate)"=w389:refnum<data-value>)  [unwired: 7 in]
                  }
                  frame "BRIGHTNESS" {
                    n110 = call-poly "Get Parameter.vi"("error in (no error)"=w396, "Stream"=w397) -> ("error out"=w395:errorcluster, "Value"=w393:i32, "Stream (duplicate)"=w394:refnum<data-value>)  [unwired: 7 in]
                  }
                  frame "CONTRAST" {
                    n111 = call-poly "Get Parameter.vi"("error in (no error)"=w401, "Stream"=w402) -> ("error out"=w400:errorcluster, "Value"=w398:i32, "Stream (duplicate)"=w399:refnum<data-value>)  [unwired: 7 in]
                  }
                  frame "SATURATION" {
                    n112 = call-poly "Get Parameter.vi"("error in (no error)"=w406, "Stream"=w407) -> ("error out"=w405:errorcluster, "Value"=w403:i32, "Stream (duplicate)"=w404:refnum<data-value>)  [unwired: 7 in]
                  }
                  frame "GAMMA" {
                    n113 = call-poly "Get Parameter.vi"("error in (no error)"=w411, "Stream"=w412) -> ("error out"=w410:errorcluster, "Value"=w408:i32, "Stream (duplicate)"=w409:refnum<data-value>)  [unwired: 7 in]
                  }
                  frame "HUE" {
                    n114 = call-poly "Get Parameter.vi"("error in (no error)"=w416, "Stream"=w417) -> ("error out"=w415:errorcluster, "Value"=w413:i32, "Stream (duplicate)"=w414:refnum<data-value>)  [unwired: 7 in]
                  }
                  frame "SHARPNESS" {
                    n115 = call-poly "Get Parameter.vi"("error in (no error)"=w421, "Stream"=w422) -> ("error out"=w420:errorcluster, "Value"=w418:i32, "Stream (duplicate)"=w419:refnum<data-value>)  [unwired: 7 in]
                  }
                  frame "BACKLIGHT_COMPENSATION" {
                    n116 = call-poly "Get Parameter.vi"("error in (no error)"=w426, "Stream"=w427) -> ("error out"=w425:errorcluster, "Value"=w423:i32, "Stream (duplicate)"=w424:refnum<data-value>)  [unwired: 7 in]
                  }
                  frame "POWER_LINE_FREQUENCY" {
                    n117 = call-poly "Get Parameter.vi"("error in (no error)"=w431, "Stream"=w432) -> ("error out"=w430:errorcluster, "Value"=w428:i32, "Stream (duplicate)"=w429:refnum<data-value>)  [unwired: 7 in]
                  }
                  frame "EXPOSURE_ABSOLUTE" {
                    n118 = call-poly "Get Parameter.vi"("error in (no error)"=w436, "Stream"=w437) -> ("error out"=w435:errorcluster, "Value"=w433:i32, "Stream (duplicate)"=w434:refnum<data-value>)  [unwired: 7 in]
                  }
                }
                n119 = property on="Dial" class="Knob (strict)"("Value"=w368) -> ()  [unwired: 2 in, 2 out]
              }
            }
            n120 = Select(t=T7."Enabled" ("Disabled"), s=w291, f=T7."Disabled and Grayed Out") -> (s? t:f=w296:T7)
            n121 = property on="Dial" class="Knob (strict)"("DisabledEnum"=w296, "Scale.Maximum"=w294, "Scale.Minimum"=w293, "Increment"=w292) -> ()  [unwired: 2 in, 2 out]
          }
          event "Dial": Value Change {
            n122 = event-data() -> ("NewVal"=w438:i32)  [unwired: 1 in, 3 out]
            n123 = case shown="\"GAIN\"" "enum" {
              tunnel: w444 -> [w452 w458 w464 w470 w476 w482 w488 w494 w500 w506 w512 w518 w524]
              tunnel: [w451 w457 w463 w469 w475 w481 w487 w493 w499 w505 w511 w517 w523] -> w443
              tunnel: w442 -> [w450 w456 w462 w468 w474 w480 w486 w492 w498 w504 w510 w516 w522]
              tunnel: [w448 w454 w460 w466 w472 w478 w484 w490 w496 w502 w508 w514 w520] -> w441
              tunnel: [w447 w453 w459 w465 w471 w477 w483 w489 w495 w501 w507 w513 w519] -> w440
              tunnel: w438 -> [w449 w455 w461 w467 w473 w479 w485 w491 w497 w503 w509 w515 w521]
              frame "FOCUS_ABSOLUTE" {
                n124 = call-poly "Set Parameter.vi"("error in (no error)"=w450, "Value"=w449, "Stream"=w452) -> ("error out"=w448:errorcluster, "Set Value"=w447:i32, "Stream (duplicate)"=w451:refnum<data-value>)  [unwired: 6 in]
              }
              frame "ZOOM_ABSOLUTE" {
                n125 = call-poly "Set Parameter.vi"("error in (no error)"=w456, "Value"=w455, "Stream"=w458) -> ("error out"=w454:errorcluster, "Set Value"=w453:i32, "Stream (duplicate)"=w457:refnum<data-value>)  [unwired: 6 in]
              }
              frame "WHITE_BALANCE_TEMPERATURE" {
                n126 = call-poly "Set Parameter.vi"("error in (no error)"=w462, "Value"=w461, "Stream"=w464) -> ("error out"=w460:errorcluster, "Set Value"=w459:i32, "Stream (duplicate)"=w463:refnum<data-value>)  [unwired: 6 in]
              }
              frame "GAIN" {
                n127 = call-poly "Set Parameter.vi"("error in (no error)"=w468, "Value"=w467, "Stream"=w470) -> ("error out"=w466:errorcluster, "Set Value"=w465:i32, "Stream (duplicate)"=w469:refnum<data-value>)  [unwired: 6 in]
              }
              frame "BRIGHTNESS" {
                n128 = call-poly "Set Parameter.vi"("error in (no error)"=w474, "Value"=w473, "Stream"=w476) -> ("error out"=w472:errorcluster, "Set Value"=w471:i32, "Stream (duplicate)"=w475:refnum<data-value>)  [unwired: 6 in]
              }
              frame "CONTRAST" {
                n129 = call-poly "Set Parameter.vi"("error in (no error)"=w480, "Value"=w479, "Stream"=w482) -> ("error out"=w478:errorcluster, "Set Value"=w477:i32, "Stream (duplicate)"=w481:refnum<data-value>)  [unwired: 6 in]
              }
              frame "SATURATION" {
                n130 = call-poly "Set Parameter.vi"("error in (no error)"=w486, "Value"=w485, "Stream"=w488) -> ("error out"=w484:errorcluster, "Set Value"=w483:i32, "Stream (duplicate)"=w487:refnum<data-value>)  [unwired: 6 in]
              }
              frame "GAMMA" {
                n131 = call-poly "Set Parameter.vi"("error in (no error)"=w492, "Value"=w491, "Stream"=w494) -> ("error out"=w490:errorcluster, "Set Value"=w489:i32, "Stream (duplicate)"=w493:refnum<data-value>)  [unwired: 6 in]
              }
              frame "HUE" {
                n132 = call-poly "Set Parameter.vi"("error in (no error)"=w498, "Value"=w497, "Stream"=w500) -> ("error out"=w496:errorcluster, "Set Value"=w495:i32, "Stream (duplicate)"=w499:refnum<data-value>)  [unwired: 6 in]
              }
              frame "SHARPNESS" {
                n133 = call-poly "Set Parameter.vi"("error in (no error)"=w504, "Value"=w503, "Stream"=w506) -> ("error out"=w502:errorcluster, "Set Value"=w501:i32, "Stream (duplicate)"=w505:refnum<data-value>)  [unwired: 6 in]
              }
              frame "BACKLIGHT_COMPENSATION" {
                n134 = call-poly "Set Parameter.vi"("error in (no error)"=w510, "Value"=w509, "Stream"=w512) -> ("error out"=w508:errorcluster, "Set Value"=w507:i32, "Stream (duplicate)"=w511:refnum<data-value>)  [unwired: 6 in]
              }
              frame "POWER_LINE_FREQUENCY" {
                n135 = call-poly "Set Parameter.vi"("error in (no error)"=w516, "Value"=w515, "Stream"=w518) -> ("error out"=w514:errorcluster, "Set Value"=w513:i32, "Stream (duplicate)"=w517:refnum<data-value>)  [unwired: 6 in]
              }
              frame "EXPOSURE_ABSOLUTE" {
                n136 = call-poly "Set Parameter.vi"("error in (no error)"=w522, "Value"=w521, "Stream"=w524) -> ("error out"=w520:errorcluster, "Set Value"=w519:i32, "Stream (duplicate)"=w523:refnum<data-value>)  [unwired: 6 in]
              }
            }
            "Set Value" <- w440
          }
          event Value Change {
            n137 = event-data() -> ("NewVal"=w525:T3)  [unwired: 1 in, 5 out]
            n138 = case shown="\"AUTO_EXPOSURE\"" "Auto Parameter" {
              tunnel: w530 -> [w537 w542 w547 w552]
              tunnel: [w536 w541 w546 w551] -> w529
              tunnel: [w535 w540 w545 w550] -> w528
              tunnel: w527 -> [w534 w539 w544 w549]
              tunnel: w525 -> [w533 w538 w543 w548]
              frame "AUTO_FOCUS" {
                n139 = call-poly "Set Automatic Parameter Mode.vi"("error in (no error)"=w534, "Automatic Parameter Mode"=w533, "Stream"=w537) -> ("error out"=w535:errorcluster, "Stream (duplicate)"=w536:refnum<data-value>)  [unwired: 7 in]
              }
              frame "AUTO_WHITEBALANCE" {
                n140 = call-poly "Set Automatic Parameter Mode.vi"("error in (no error)"=w539, "Automatic Parameter Mode"=w538, "Stream"=w542) -> ("error out"=w540:errorcluster, "Stream (duplicate)"=w541:refnum<data-value>)  [unwired: 7 in]
              }
              frame "AUTO_GAIN" {
                n141 = call-poly "Set Automatic Parameter Mode.vi"("error in (no error)"=w544, "Automatic Parameter Mode"=w543, "Stream"=w547) -> ("error out"=w545:errorcluster, "Stream (duplicate)"=w546:refnum<data-value>)  [unwired: 7 in]
              }
              frame "AUTO_EXPOSURE" {
                n142 = call-poly "Set Automatic Parameter Mode.vi"("error in (no error)"=w549, "Automatic Parameter Mode"=w548, "Stream"=w552) -> ("error out"=w550:errorcluster, "Stream (duplicate)"=w551:refnum<data-value>)  [unwired: 7 in]
              }
            }
          }
          event "Erase": Value Change {
            n143 = event-data() -> ()  [unwired: 1 in, 1 out]
            n144 = property on="2D Picture" class="Pict"("Erase First"=u8 1) -> ()  [unwired: 2 in, 2 out]
          }
          event "Picture Zoom": Value Change {
            n145 = event-data() -> ("NewVal"=w561:dbl)  [unwired: 1 in]
            n146 = property on="2D Picture" class="Pict"(error in=w560, "ZoomFactor"=w561) -> (error out=w559:errorcluster)  [unwired: 1 in, 1 out]
          }
        }
        n147 = Or(x=w26, y=w24) -> (x .or. y?=w25:bool)
      }
    }
    frame Error {
    }
  }
  n148 = Delete Data Value Reference(data value reference=w7) -> ()  [unwired: 1 in, 2 out]
  n149 = call "Destroy.vi"("CameraManager"=w12) -> ()  [unwired: 10 in, 1 out]
  n150 = call <vilib>:"Simple Error Handler.vi"("error in (no error)"=w6) -> ()  [unwired: 4 in, 5 out]
